vi "test Receive Stop Flag.vi"(8 "error in (no error)":errorcluster, 11 "TestCase in":refnum<class "Test TCP Stream Transmission.lvclass">) -> (0 "error out":errorcluster, 3 "TestCase out":refnum<class "Test TCP Stream Transmission.lvclass">)   [LabVIEW 2020, in "Test TCP Stream Transmission.lvclass"]
uses:
  Test TCP Stream Transmission.lvclass
  <vilib>/addons/_JKI Toolkits/VI Tester/TestCase.llb/TestCase.lvclass
  Source/Protocols/TCP Strategy/TCP Stream Initiator/TCP Stream Initiator.lvclass
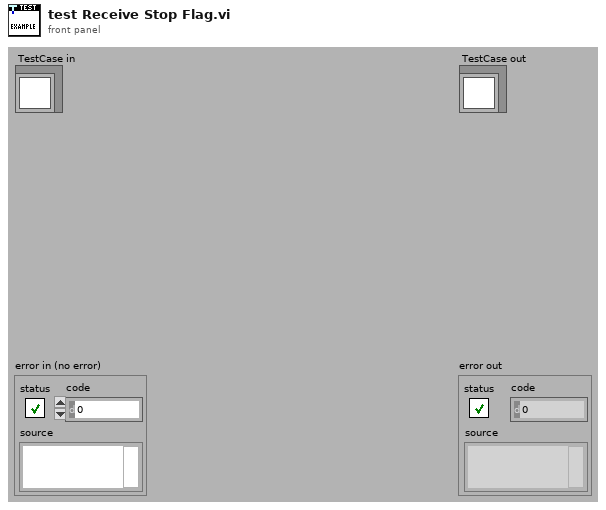
[diagram p1: front panel]
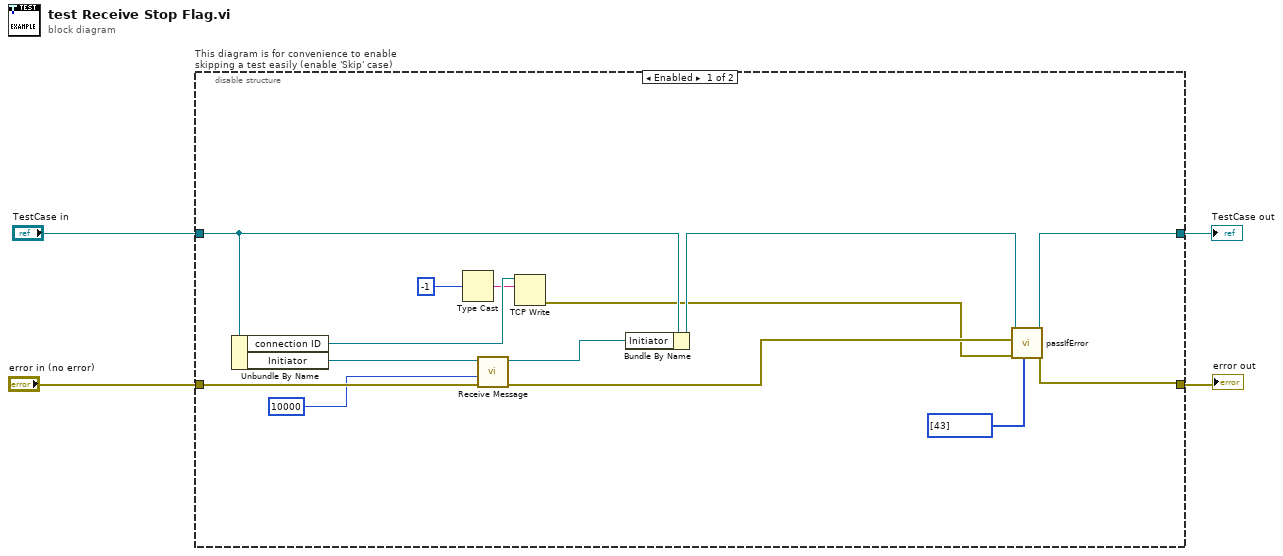
[diagram p0: block diagram]
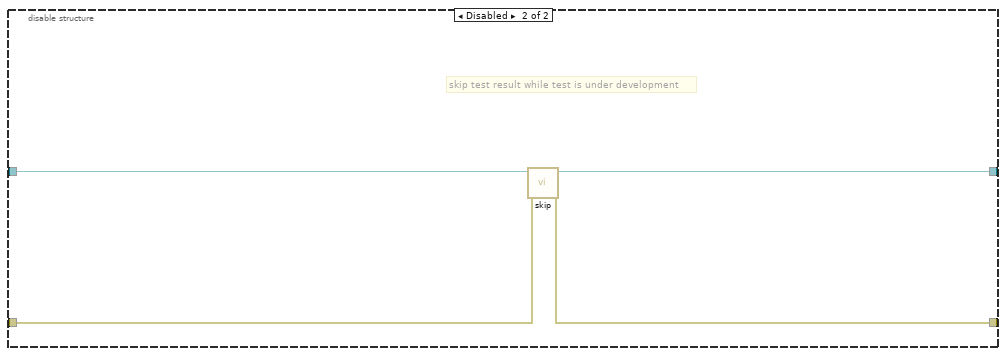
[diagram p2: hidden frame]
diagram:
  n1 = disable-structure "This diagram is for convenience to enable skipping a test easily (enable 'Skip' case)" shown="Enabled" {
    disable-tunnel: "TestCase in" -> [w13 w22]
    disable-tunnel: [w18 w20] -> w1
    disable-tunnel: [w17 w21] -> w3
    disable-tunnel: "error in (no error)" -> [w16 w19]
    frame Enabled {
      n2 = Unbundle By Name(w13) -> ("connection ID"=w10:refnum<k5>, "Initiator"=w15:refnum<class "TCP Stream Initiator.lvclass">)
      n3 = Type Cast(x=-1 ("length")) -> (*(type *) &x=w9:string)  [unwired: 1 in]
      n4 = call-dynamic "Receive Message.vi"("error in (no error)"=w16, "timeout ms (-1)"=10000, "TCP Stream in"=w15) -> ("error out"=w7:errorcluster, "TCP Stream out"=w14:refnum<class "TCP Stream Initiator.lvclass">)  [unwired: 4 in, 3 out]
      n5 = TCP Write(connection ID=w10, data in=w9) -> (error out=w5:errorcluster)  [unwired: 2 in, 2 out]
      n6 = Bundle By Name(cluster=w13, "Initiator"=w14) -> (w12:refnum<class "Test TCP Stream Transmission.lvclass">)
      n7 = call-dynamic "passIfError.vi"("passing error codes (default = any error code)"=i32[] [43], "error in (no error)"=w5, "error"=w7, "TestCase in"=w12) -> ("error out"=w17:errorcluster, "TestCase out"=w18:refnum<class "Test TCP Stream Transmission.lvclass">)  [unwired: 6 in]
    }
    frame Disabled {
      # "skip test result while test is under development"
      n8 = call <vilib>:"skip.vi"("error in (no error)"=w19, "TestCase in"=w22) -> ("error out"=w21:errorcluster, "TestCase out"=w20:refnum<class "Test TCP Stream Transmission.lvclass">)  [unwired: 8 in]
    }
  }
  "error out" <- w3
  "TestCase out" <- w1
